vi "Get Washing Cluster Array.vi"(10 "all rows":i64[][](array[numeric]), 11 "Wash Options":T1) -> (3 "Array":T2[](array[typedef]))   [LabVIEW 2024]
uses:
  Washing Control Cluster.ctl
  States of Washing.ctl
  Controls/Wash Options.ctl
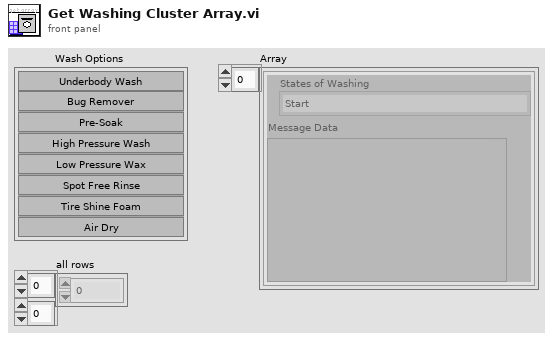
[diagram p1: front panel]
types:
  T1 = typedef "Wash Options.ctl" = cluster{"Underbody Wash":bool, "Bug Remover":bool, "Pre-Soak":bool, "High Pressure Wash":bool, "Low Pressure Wax":bool, "Spot Free Rinse":bool, "Tire Shine Foam":bool, "Air Dry":bool}
  T2 = typedef "Washing Control Cluster.ctl" = cluster{"Message Data":variant, "States of Washing":T3}
  T3 = typedef "States of Washing.ctl" = enum16{"Start", "Under Body Wash", "Bug Remover", "Pre-Soak", "High Pressure Wax", "Low Pressure Wax", "Spot Free Rinse", "Tire Shine Foam", "Air Dry", "End", "Initialize"}
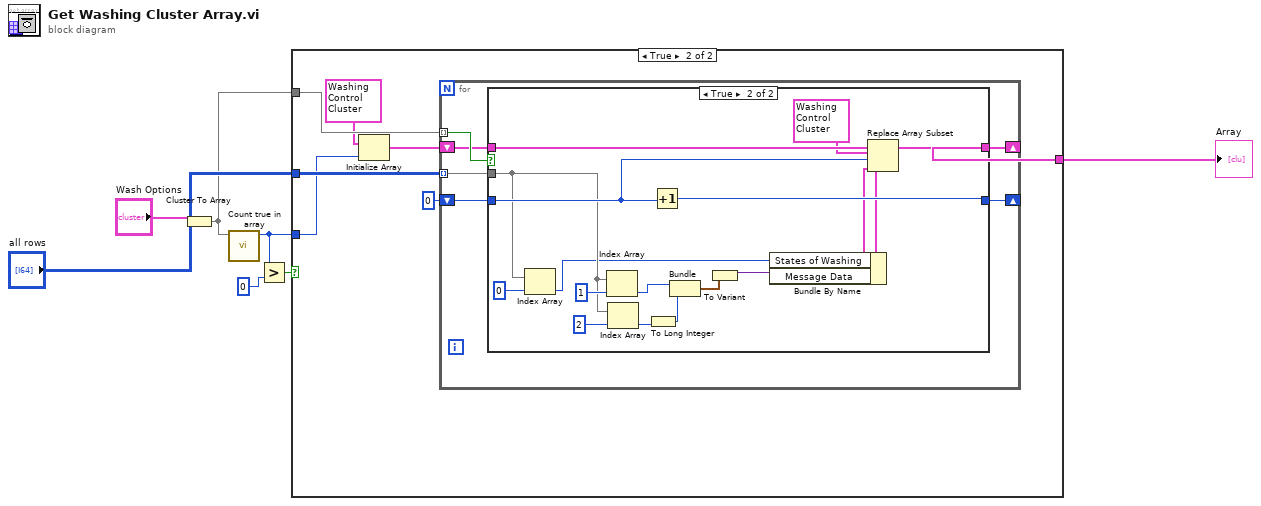
[diagram p0: block diagram]
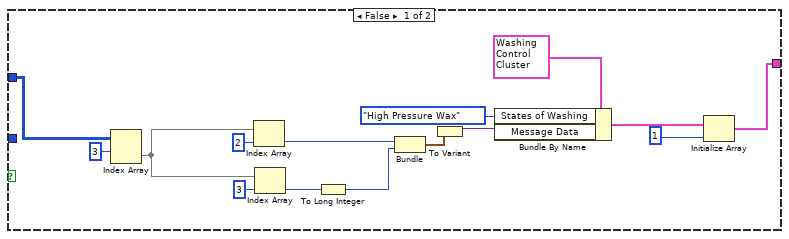
[diagram p2: hidden frame]
diagram:
  n1 = Cluster To Array(cluster="Wash Options") -> (array=w6:bool[])
  n2 = call "Count true in array.vi"("Wash Options"=w6) -> ("Numeric"=w3:i32)  [unwired: 10 in]
  n3 = Greater?(x=w3, y=0) -> (0:w1:bool)
  n4 = case shown="True" w1 {
    tunnel: "all rows" -> [w21 w27]
    tunnel: w6 -> [_ w26]
    tunnel: w3 -> [_ w24]
    tunnel: [w9 w23] -> w4
    frame False {
      n5 = Index Array(array=w21, index (row)=3) -> (element=w15:i64[])  [unwired: 1 in]
      n6 = Index Array(array=w15, index=2 ("index (row)")) -> (element=w14:i64)
      n7 = Index Array(array=w15, index=3 ("index (row)")) -> (element=w13:i64)
      n8 = To Long Integer(number=w13) -> (32bit integer=w12:i32)
      n9 = Bundle("Numeric"=w14, w12) -> (w19:cluster{"Numeric":i64, i32})  [unwired: 1 in]
      n10 = To Variant(anything=w19) -> (Variant=w18:variant)
      n11 = Bundle By Name(cluster=T2 {"Message Data"=variant, "States of Washing"=enum."Start"} ("Washing Control Cluster"), "States of Washing"=States_of_Washing."High Pressure Wax", "Message Data"=w18) -> (w10:T2)
      n12 = Initialize Array(w10, 1 ("dimension size")) -> (w9:T2[])
    }
    frame True {
      n13 = Initialize Array(T2 {"Message Data"=variant, "States of Washing"=enum."Start"} ("Washing Control Cluster"), w24) -> (w29:T2[])
      n14 = for {
        tunnel: w26 -> [w35] mode=indexing
        tunnel: w27 -> [w31] mode=indexing
        shift-right: [w33] -> _
        shift-left: u16 0 -> [w34]
        shift-right: [w30] -> w23
        shift-left: w29 -> [w32]
        n15 = case shown="True" w35 {
          tunnel: [w37 w53] -> w33
          tunnel: w34 -> [w37 w52]
          tunnel: w32 -> [w36 w51]
          tunnel: w31 -> [_ w39]
          tunnel: [w36 w43] -> w30
          frame False {
          }
          frame True {
            n16 = Index Array(array=w39, index=0) -> (element=w38:i64)
            n17 = Index Array(array=w39, index=1) -> (element=w48:i64)
            n18 = Index Array(array=w39, index=2) -> (element=w42:i64)
            n19 = To Long Integer(number=w42) -> (32bit integer=w41:i32)
            n20 = Increment(x=w52) -> (x+1=w53:u16)
            n21 = Bundle("Numeric"=w48, w41) -> (w47:cluster{"Numeric":i64, i32})  [unwired: 1 in]
            n22 = To Variant(anything=w47) -> (Variant=w45:variant)
            n23 = Bundle By Name(cluster=T2 {"Message Data"=variant, "States of Washing"=enum."Start"} ("Washing Control Cluster"), "States of Washing"=w38, "Message Data"=w45) -> (w44:T2)
            n24 = Replace Array Subset(array=w51, new element=w44, index=w52) -> (w43:T2[])
          }
        }
      }
    }
  }
  "Array" <- w4
